vi "Thev-L to Z (1D).vi"(2 "L (mm)":dbl[](array[numeric]) format="%#_13g", 3 "Frequency (Hz)":dbl[](array[numeric])) -> (0 "Zx":cdb[][](array[numeric]))   [LabVIEW 2015]
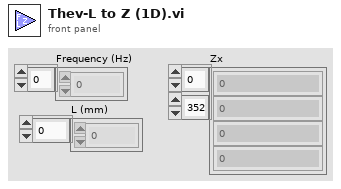
[diagram p1: front panel]
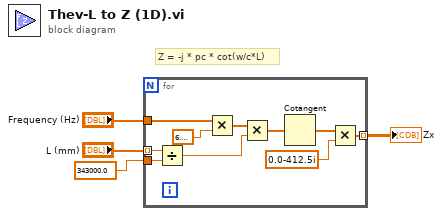
[diagram p0: block diagram]
diagram:
  # "Z = -j * pc * cot(w/c*L)"
  n1 = for {
    tunnel: "Frequency (Hz)" -> [w14]
    tunnel: 343000.0 ("y") -> [w9]
    tunnel: [w6] -> w1 mode=indexing
    tunnel: "L (mm)" -> [w5] mode=indexing
    n2 = Divide(x=w5, y=w9) -> (x/y=w10:dbl)
    n3 = Multiply(x=w14, y=6.283185307179586) -> (x*y=w8:dbl[])
    n4 = Multiply(x=w8, y=w10) -> (x*y=w11:dbl[])
    n5 = Cotangent(1:w11) -> (0:w12:dbl[])
    n6 = Multiply(x=w12, y=cdb 0.0-412.5i) -> (x*y=w6:cdb[])
  }
  "Zx" <- w1
